vi "ma_Force Restart no State.vi"(6 "state info":T2 {"real spectrum" format="%0.2f"; "averages completed" format="%0.2f"; "df" format="%0.2f"; "complex spectrum" format="%0.2f"; "spectrum parameters"."window" items=["Rectangle"=0, "Hanning"=1, "Hamming"=2, "Blackman-Harris"=3, "Exact Blackman"=4, "Blackman"=5, "Flat Top"=6, "4 Term B-Harris "=7, "7 Term B-Harris"=8, "Low Sidelobe"=9, "Blackman Nuttall"=11, "Triangle"=30, "Bartlett-Hanning"=31, "Bohman"=32, "Parzen"=33, "Welch"=34, "Kaiser"=60, "Dolph-Chebyshev"=61, "Gaussian"=62]; "dt" format="%0.2f"; "timestamp" format="%0.2f"; "dt history" format="%0.2f"; "t0 history" format="%0.2f"}, 7 "caller VI name":string, 8 "force restart averaging in":bool, 9 "restart averaging (F)":bool, 10 "window":T1=1 items=["Rectangle"=0, "Hanning"=1, "Hamming"=2, "Blackman-Harris"=3, "Exact Blackman"=4, "Blackman"=5, "Flat Top"=6, "4 Term B-Harris "=7, "7 Term B-Harris"=8, "Low Sidelobe"=9, "Blackman Nuttall"=11, "Triangle"=30, "Bartlett-Hanning"=31, "Bohman"=32, "Parzen"=33, "Welch"=34, "Kaiser"=60, "Dolph-Chebyshev"=61, "Gaussian"=62], 11 "averaging parameters":T3={"averaging mode"=enum."No averaging", "weighting mode"=enum."Exponential", "number of averages"=10} {"number of averages" min=1}) -> (0 "error out":errorcluster, 1 "retrieve last spectrum":bool, 2 "force restart averaging":bool, 3 "skip processing":errorcluster, 4 "state info":T2 {"real spectrum" format="%0.2f"; "averages completed" format="%0.2f"; "df" format="%0.2f"; "complex spectrum" format="%0.2f"; "spectrum parameters"."window" items=["Rectangle"=0, "Hanning"=1, "Hamming"=2, "Blackman-Harris"=3, "Exact Blackman"=4, "Blackman"=5, "Flat Top"=6, "4 Term B-Harris "=7, "7 Term B-Harris"=8, "Low Sidelobe"=9, "Blackman Nuttall"=11, "Triangle"=30, "Bartlett-Hanning"=31, "Bohman"=32, "Parzen"=33, "Welch"=34, "Kaiser"=60, "Dolph-Chebyshev"=61, "Gaussian"=62]; "dt" format="%0.2f"; "timestamp" format="%0.2f"; "dt history" format="%0.2f"; "t0 history" format="%0.2f"})   [LabVIEW 2020, in "NI_MAPro.lvlib"]
uses:
  NI_MAPro.lvlib
  windowTd.ctl
  NI_AALPro.lvlib
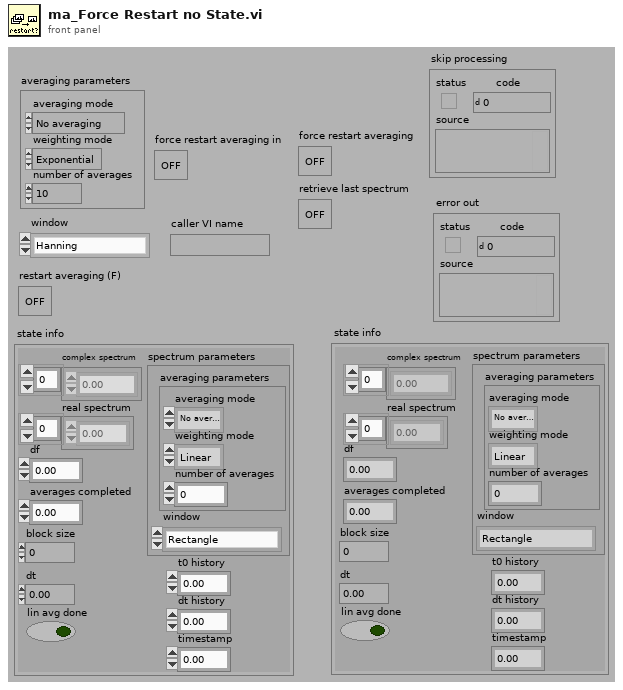
[diagram p1: front panel]
types:
  T1 = typedef "NI_AALPro.lvlib/windowTd.ctl" = u32
  T2 = cluster{"block size":i32, "dt":dbl, "spectrum parameters":cluster{"averaging parameters":cluster{"averaging mode":enum16{"No averaging", "Vector averaging", "RMS averaging", "Peak hold"}, "weighting mode":enum16{"Linear", "Exponential"}, "number of averages":u32}, "window":T1}, "df":dbl, "averages completed":dbl, "complex spectrum":cdb[], "real spectrum":dbl[], "t0 history":dbl, "dt history":dbl, "timestamp":dbl, "lin avg done":bool}
  T3 = cluster{"averaging mode":enum16{"No averaging", "Vector averaging", "RMS averaging", "Peak hold"}, "weighting mode":enum16{"Linear", "Exponential"}, "number of averages":u32}
  T4 = cluster{"averaging parameters":cluster{"averaging mode":enum16{"No averaging", "Vector averaging", "RMS averaging", "Peak hold"}, "weighting mode":enum16{"Linear", "Exponential"}, "number of averages":u32}, "window":T1}
  T5 = enum16{"No averaging", "Vector averaging", "RMS averaging", "Peak hold"}
  T6 = cluster{"status":bool, "code":i32, "caller VI name":string}
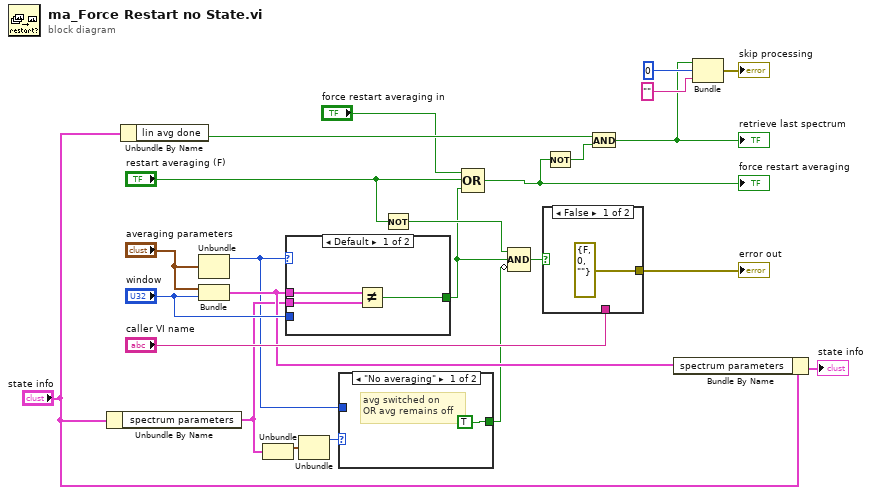
[diagram p0: block diagram]
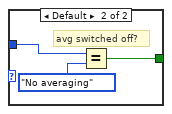
[diagram p2: hidden frame]
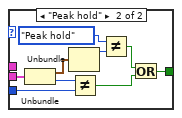
[diagram p3: hidden frame]
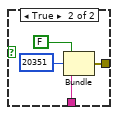
[diagram p4: hidden frame]
diagram:
  n1 = Unbundle By Name("state info") -> ("spectrum parameters"=w7:T4)
  n2 = Unbundle By Name("state info") -> ("lin avg done"=w12:bool)
  n3 = Unbundle("averaging parameters") -> ("averaging mode"=w5:T5)  [unwired: 2 out]
  n4 = Bundle("averaging parameters"="averaging parameters", "window"="window") -> (w15:T4)  [unwired: 1 out]
  n5 = Unbundle(w7) -> ("averaging parameters"=w8:T3)  [unwired: 1 out]
  n6 = case shown="Default" w5 {
    tunnel: w7 -> [w27 w36]
    tunnel: [w26 w30] -> w3
    tunnel: w15 -> [w25 _]
    tunnel: "window" -> [_ w34]
    frame Default {
      n7 = Not Equal?(x=w25, y=w27) -> (x != y?=w26:bool)
    }
    frame "Peak hold" {
      n8 = Unbundle(w36) -> ("averaging parameters"=w33:T3, "window"=w35:T1)
      n9 = Unbundle(w33) -> ("averaging mode"=w29:T5)  [unwired: 2 out]
      n10 = Not Equal?(x=w35, y=w34) -> (x != y?=w31:bool)
      n11 = Not Equal?(x=T5."Peak hold" ("y"), y=w29) -> (x != y?=w32:bool)
      n12 = Or(x=w32, y=w31) -> (x .or. y?=w30:bool)
    }
  }
  n13 = Unbundle(w8) -> ("averaging mode"=w6:T5)  [unwired: 2 out]
  n14 = case shown="\"No averaging\"" w6 {
    tunnel: w5 -> [_ w40]
    tunnel: [TRUE w38] -> w2
    frame "No averaging" {
      # "avg switched on \nOR avg remains off"
    }
    frame Default {
      # "avg switched off?"
      n15 = Equal?(x=w40, y=T5."No averaging" ("averaging mode")) -> (x = y?=w38:bool)
    }
  }
  n16 = Not(x="restart averaging (F)") -> (.not. x?=w4:bool)
  n17 = Compound Arithmetic op=OR("force restart averaging in", "restart averaging (F)", w3) -> (w9:bool)
  "force restart averaging" <- w9
  n18 = Compound Arithmetic op=AND(w4, w3, invert w2) -> (w1:bool)
  n19 = case shown="False" w1 {
    tunnel: [errorcluster {"status"=FALSE, "code"=0, "source"=""} ("error out") w45] -> w20
    tunnel: "caller VI name" -> [_ w42]
    frame False {
    }
    frame True {
      n20 = Bundle("status"=FALSE, "code"=20351, "caller VI name"=w42) -> (w45:T6)  [unwired: 1 out]
    }
  }
  "error out" <- w20
  n21 = Not(x=w9) -> (.not. x?=w14:bool)
  n22 = And(x=w12, y=w14) -> (x .and. y?=w21:bool)
  "retrieve last spectrum" <- w21
  n23 = Bundle By Name(cluster="state info", "spectrum parameters"=w15) -> (→"state info":T2)
  n24 = Bundle(w21, "code"=0, "source"="") -> (→"skip processing":cluster{bool, "code":i32, "source":string})  [unwired: 1 out]
